vi "Entry.vi"(8 "error in (no error)":errorcluster, 11 "Ready in":refnum<class "Ready.lvclass">) -> (0 "error out":errorcluster, 3 "Ready out":refnum<class "Ready.lvclass">)   [LabVIEW 2014, in "States.lvlib" / "Ready.lvclass"]
doc: "This override sends a Log Event message to the UI, with the string \"Entering Idle State\" as its payload."
uses:
  Ready.lvclass
  Process State/CoordinatorState.lvclass
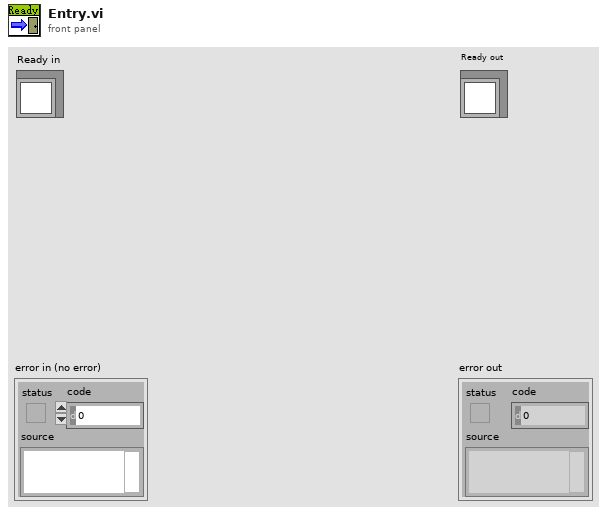
[diagram p1: front panel]
types:
  T1 = enum32{"Joy", "Map", "Voice", "Input", "Undefined"}
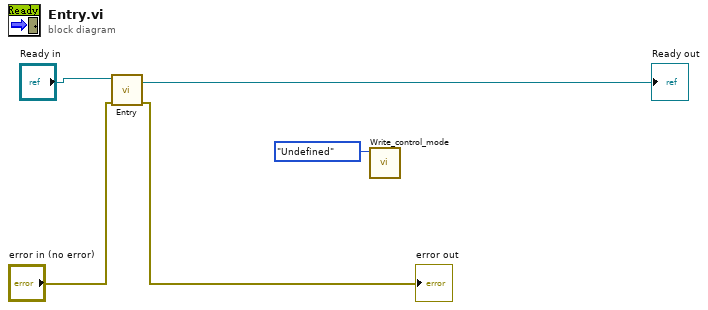
[diagram p0: block diagram]
diagram:
  n1 = call-parent "Entry.vi"("error in (no error)"="error in (no error)", "New State"="Ready in") -> ("error out"=→"error out":errorcluster, "State out"=→"Ready out":refnum<class "Ready.lvclass">)  [unwired: 8 in]
  n2 = call "Write_control_mode.vi"("Control_Mode"=T1."Undefined") -> ()  [unwired: 11 in]
